vi "PWM Set Pulse.vi"(9 "pPulse":u16[](array[numeric])=[0, 0, 0, 0, 0, 0, 0, 0], 10 "ChannelMask":u8, 11 "DevHandle":i32) -> (1 "pPulse out":u16[](array[numeric]), 3 "function return":i32)   [LabVIEW 2010, in "usb2pwm.lvlib"]
doc: "int WINAPI PWM_SetPulse(int DevHandle,unsigned char ChannelMask,unsigned short *pPulse);"
uses:
  usb2pwm.lvlib
  USB2XXX/trunk/USB2XXX/USB2XXX/vs2019/Release/USB2XXX.dll
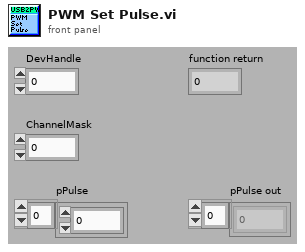
[diagram p1: front panel]
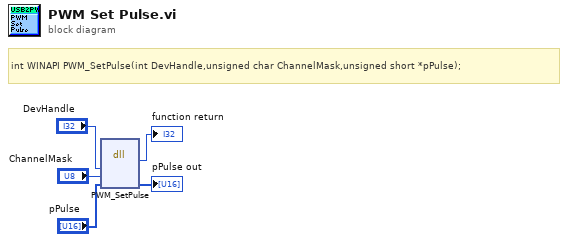
[diagram p0: block diagram]
diagram:
  # "int WINAPI PWM_SetPulse(int DevHandle,unsigned char ChannelMask,unsigned short *pPulse);"
  n1 = dll-call lib="E:/Projects/USB2XXX/trunk/USB2XXX/USB2XXX/vs2019/Release/USB2XXX.*" fn="PWM_SetPulse"("DevHandle"="DevHandle", "ChannelMask"="ChannelMask", "pPulse"="pPulse") -> (→"function return":i32, "pPulse"=→"pPulse out":u16[])  [unwired: 5 in, 2 out]
